vi "Format EbsInstanceBlockDeviceMappingResponseType_LVXML.vi"(8 "error in (no error)":errorcluster, 10 "xmlData in":T2, 11 "AWS_EC2 in":refnum<class "AWS_EC2.lvclass">) -> (0 "error out":errorcluster, 2 "EbsInstanceBlockDeviceMappingResponseType":T3, 3 "AWS_EC2 out":refnum<class "AWS_EC2.lvclass">)   [LabVIEW 2014, in "AWS_EC2.lvlib" / "AWS_EC2.lvclass"]
uses:
  AWS_EC2.lvclass
  EC2 Datatypes/EbsInstanceBlockDeviceMappingResponseType.ctl
  lv-xml-parser/r0/trunk/VI Source/EventType.ctl
  AWS_EC2.lvlib
  lv-xml-parser/r0/trunk/VI Source/LV XML Parser.lvlib
  AWS Core Lib/VI Source/AWS_Core.lvlib
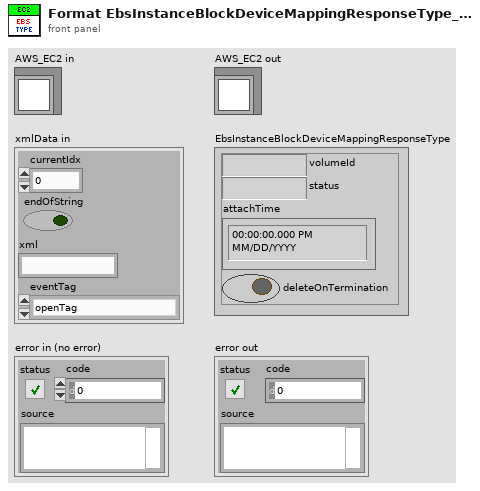
[diagram p1: front panel]
types:
  T1 = typedef "LV XML Parser.lvlib/EventType.ctl" = enum16{"openTag", "endOpenTag", "closeTag", "comment", "endComment", "endOfFile", "attribute", "startXml"}
  T2 = cluster{"currentIdx":i32, "endOfString":bool, "xml":string, "eventTag":T1}
  T3 = typedef "AWS_EC2.lvlib/EbsInstanceBlockDeviceMappingResponseType.ctl" = cluster{"volumeId":string, "status":string, "attachTime":timestamp, "deleteOnTermination":bool}
  T4 = cluster{"namespaceUri":string, "localName":string}
  T5 = cluster{"Attributes":cluster{"localName":string, "namespaceUri":string, "value":string}[], "localName":string, "namespaceUri":string, "valueXmlData":cluster{"currentIdx":i32, "endOfString":bool, "xml":string, "eventTag":T1}}[]
  T6 = cluster{"Attributes":cluster{"localName":string, "namespaceUri":string, "value":string}[], "localName":string, "namespaceUri":string, "valueXmlData":cluster{"currentIdx":i32, "endOfString":bool, "xml":string, "eventTag":T1}}
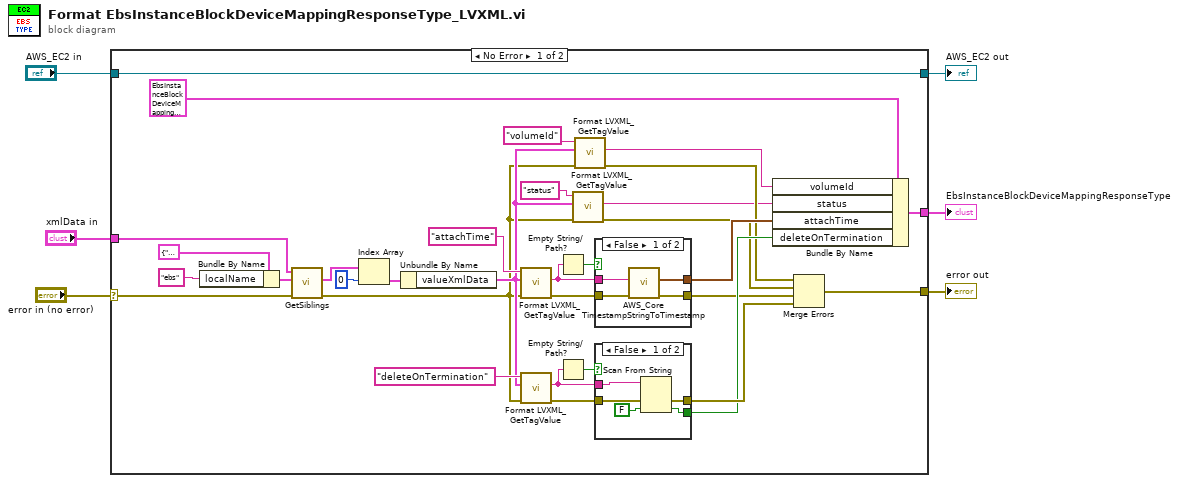
[diagram p0: block diagram]
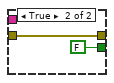
[diagram p2: hidden frame]
diagram:
  n1 = case shown="No Error" "error in (no error)" {
    selector: "error in (no error)" -> [w31 w52]
    tunnel: "xmlData in" -> [w32 _]
    tunnel: [w15 w52] -> w2
    tunnel: [w29 _] -> w4
    tunnel: [w7 w51] -> w5
    tunnel: "AWS_EC2 in" -> [w7 w51]
    frame No Error {
      n2 = Bundle By Name(cluster=T4 {"namespaceUri"="", "localName"=""} ("limitToTag"), "localName"="ebs" ("Tag name")) -> (w37:T4)
      n3 = call "GetSiblings.vi"("error in (no error)"=w31, "limitToTag"=w37, "xmlData"=w32) -> ("error out"=w23:errorcluster, "Siblings"=w34:T5)  [unwired: 7 in]
      n4 = Index Array(array=w34, index=0) -> (element=w33:T6)
      n5 = Unbundle By Name(w33) -> ("valueXmlData"=w24:T2)
      n6 = call "Format LVXML_GetTagValue.vi"("error in (no error)"=w23, "xmlDataIn"=w24, "Tag name"="attachTime") -> ("error out"=w16:errorcluster, "Value"=w21:string)  [unwired: 6 in, 1 out]
      n7 = call "Format LVXML_GetTagValue.vi"("error in (no error)"=w23, "xmlDataIn"=w24, "Tag name"="deleteOnTermination") -> ("error out"=w17:errorcluster, "Value"=w18:string)  [unwired: 6 in, 1 out]
      n8 = Empty String/Path?(string/path=w21) -> (empty?=w22:bool)
      n9 = Empty String/Path?(string/path=w18) -> (empty?=w19:bool)
      n10 = call "Format LVXML_GetTagValue.vi"("error in (no error)"=w23, "xmlDataIn"=w24, "Tag name"="status") -> ("error out"=w10:errorcluster, "Value"=w8:string)  [unwired: 6 in, 1 out]
      n11 = call "Format LVXML_GetTagValue.vi"("error in (no error)"=w23, "xmlDataIn"=w24, "Tag name"="volumeId") -> ("error out"=w11:errorcluster, "Value"=w12:string)  [unwired: 6 in, 1 out]
      n12 = case shown="False" w22 {
        tunnel: w21 -> [w49 _]
        tunnel: [w48 _] -> w20
        tunnel: w16 -> [w47 w50]
        tunnel: [w46 w50] -> w9
        frame False {
          n13 = call "AWS_Core TimestampStringToTimestamp.vi"("error in"=w47, "AWS Timestamp String"=w49) -> ("error out"=w46:errorcluster, "Time Stamp Control"=w48:timestamp)  [unwired: 8 in]
        }
        frame True {
        }
      }
      n14 = case shown="False" w19 {
        tunnel: [w43 w45] -> w14
        tunnel: [w42 FALSE] -> w13
        tunnel: w17 -> [w40 w45]
        tunnel: w18 -> [w39 _]
        frame False {
          n15 = Scan From String(input string=w39, error in=w40, default 1=FALSE) -> (error out=w43:errorcluster, output 1=w42:bool)  [unwired: 2 in, 2 out]
        }
        frame True {
        }
      }
      n16 = Bundle By Name(cluster=T3 {"volumeId"="", "status"="", "attachTime"=timestamp(0 s since 1904-01-01), "deleteOnTermination"=FALSE} ("EbsInstanceBlockDeviceMappingResponseType"), "volumeId"=w12, "status"=w8, "attachTime"=w20, "deleteOnTermination"=w13) -> (w29:T3)
      n17 = Merge Errors(w11, w10, w9, w14) -> (w15:errorcluster)
    }
    frame Error {
    }
  }
  "AWS_EC2 out" <- w5
  "EbsInstanceBlockDeviceMappingResponseType" <- w4
  "error out" <- w2
